vi "RemoveByIndex.vi"(8 "error in (no error)":errorcluster, 10 "Index":i32, 11 "Collection in":refnum<class "CollectionByValue.lvclass">) -> (0 "error out":errorcluster, 1 "found":bool, 2 "LabVIEW Object Removed":refnum<class>, 3 "Collection out":refnum<class "CollectionByValue.lvclass">, 4 "Name":string)   [LabVIEW 2021, in "Collection.lvlib" / "CollectionByValue.lvclass"]
uses:
  CollectionByValue.lvclass
  CollectionByValue.lvclass/CollectionByValue.ctl
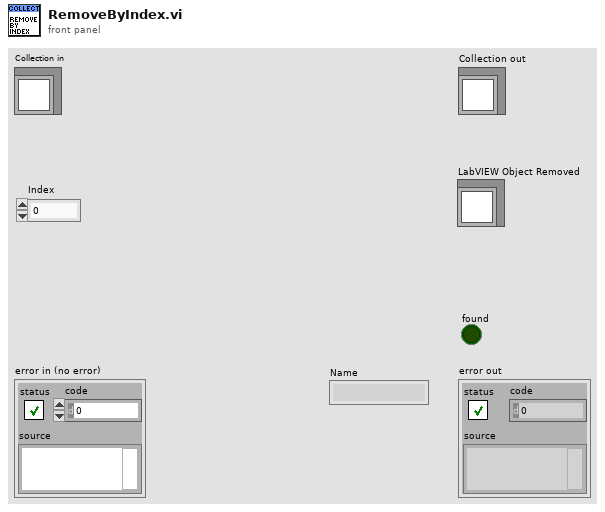
[diagram p1: front panel]
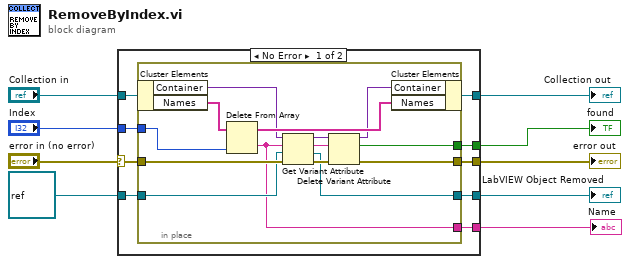
[diagram p0: block diagram]
diagram:
  n1 = case shown="No Error" "error in (no error)" {
    selector: "error in (no error)" -> [w14 w34]
    tunnel: [w13 w34] -> w8
    tunnel: [w17 w33] -> w6
    tunnel: "Collection in" -> [w18 w33]
    tunnel: "Index" -> [w16 _]
    tunnel: [w15 _] -> w4
    tunnel: [w12 w32] -> w2
    tunnel: refnum<class> refnum ("LabVIEW Object") -> [w11 w32]
    tunnel: [w10 _] -> w1
    frame No Error {
      n2 = in-place {
        in-place-border: w16 -> [w22]
        in-place-border: [w29] -> w15
        in-place-border: w14 -> [w26]
        in-place-border: [w28] -> w13
        in-place-border: [w21] -> w12
        in-place-border: w11 -> [w20]
        in-place-border: [w19] -> w10
        n3 = in-place-cluster #1(w18) -> ("Container"=w24:variant, "Names"=w31:string[])
        n4 = Delete From Array(array=w31, index=w22) -> (deleted portion=w19:string, array with subset deleted=w30:string[])  [unwired: 1 in]
        n5 = Get Variant Attribute(Variant=w24, name=w19, default value (empty Variant)=w20, error in=w26) -> (duplicate Variant=w23:variant, value=w21:refnum<class>, error out=w25:errorcluster)  [unwired: 1 out]
        n6 = Delete Variant Attribute(4:w25, 6:w19, 7:w23) -> (0:w28:errorcluster, 2:w29:bool, 3:w27:variant)
        n7 = in-place-cluster #1("Container"=w27, "Names"=w30) -> (w17:refnum<class "CollectionByValue.lvclass">)
      }
    }
    frame Error {
    }
  }
  "error out" <- w8
  "Collection out" <- w6
  "found" <- w4
  "LabVIEW Object Removed" <- w2
  "Name" <- w1
